vi "SQLite Editing Tests.vi"(8 "Error In (no error)":errorcluster) -> (0 "Error Out":errorcluster)   [LabVIEW 2023]
uses:
  SQLite DB Operator/SQLite DB Operator.lvclass
  H:/Desktop/LabVIEW/LabView Repo/Expenses-Tracker-DB-Operator/DB Operator/DB Operator.lvclass
  SQLite DB Operator/SQLite DB Operator.lvclass/SQLite DB Operator.ctl
  <vilib>/drjdpowell/SQLite Library/SQL Connection/Execute SQL (No results).vi
  <vilib>/drjdpowell/SQLite Library/SQL Connection/Connection.lvclass
  <vilib>/drjdpowell/SQLite Library/SQLite.lvlib
  <vilib>/addons/_JKI Toolkits/Caraya/classes/Test/Test.lvclass
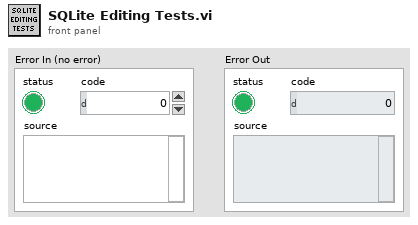
[diagram p1: front panel]
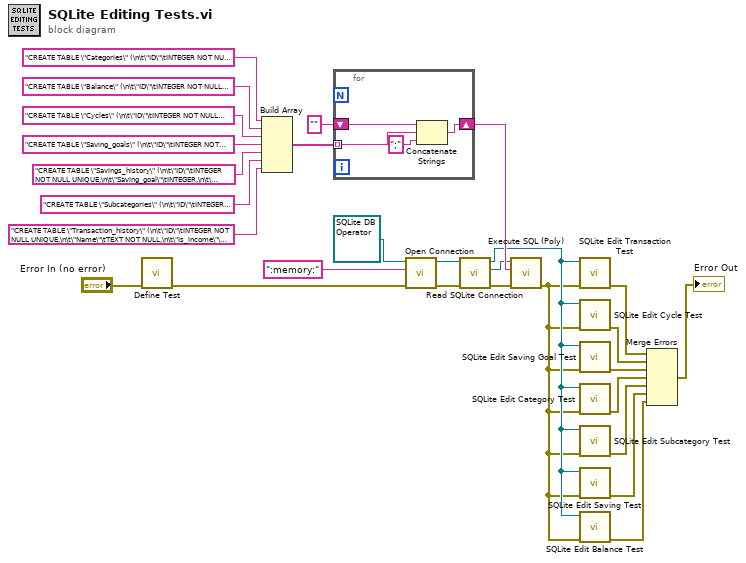
[diagram p0: block diagram]
diagram:
  n1 = call <vilib>:"Define Test.vi"("error in (no error)"="Error In (no error)") -> ("error out"=w11:errorcluster)  [unwired: 9 in, 1 out]
  n2 = Build Array("CREATE TABLE \"Categories\" (\n\t\"ID\"\tINTEGER NOT NULL UNIQUE,\n\t\"Name\"\tTEXT,\n\tPRIMARY KEY(\"ID\" AUTOINCREMENT)\n)", "CREATE TABLE \"Balance\" (\n\t\"ID\"\tINTEGER NOT NULL UNIQUE,\n\t\"Value\"\tREAL NOT NULL,\n\t\"Last_update\"\tINTEGER NOT NULL,\n\tPRIMARY KEY(\"ID\" AUTOINCREMENT)\n)", "CREATE TABLE \"Cycles\" (\n\t\"ID\"\tINTEGER NOT NULL UNIQUE,\n\t\"Name\"\tTEXT,\n\t\"Day_of_occurence\"\tINTEGER,\n\t\"Description\"\tTEXT,\n\tPRIMARY KEY(\"ID\" AUTOINCREMENT)\n)", "CREATE TABLE \"Saving_goals\" (\n\t\"ID\"\tINTEGER NOT NULL UNIQUE,\n\t\"Is_active\"\tINTEGER NOT NULL,\n\t\"Name\"\tTEXT,\n\t\"Current_value\"\tREAL NOT NULL,\n\t\"Target_value\"\tREAL NOT NULL,\n\t\"Date_of_entry\"\tINTEGER NOT NULL,\n\t\"Due_date\"\tINTEGER,\n\t\"Last_update\"\tINTEGER NOT NULL,\n\t\"Description\"\tTEXT,\n\tPRIMARY KEY(\"ID\" AUTOINCREMENT)\n)", "CREATE TABLE \"Savings_history\" (\n\t\"ID\"\tINTEGER NOT NULL UNIQUE,\n\t\"Saving_goal\"\tINTEGER,\n\t\"Value\"\tINTEGER NOT NULL,\n\t\"Date_of_entry\"\tINTEGER NOT NULL,\n\t\"Description\"\tTEXT,\n\tFOREIGN KEY(\"Saving_goal\") REFERENCES \"Saving_goals\"(\"ID\") ON DELETE RESTRICT,\n\tPRIMARY KEY(\"ID\" AUTOINCREMENT)\n)", "CREATE TABLE \"Subcategories\" (\n\t\"ID\"\tINTEGER NOT NULL UNIQUE,\n\t\"Name\"\tTEXT,\n\t\"Category\"\tINTEGER,\n\tFOREIGN KEY(\"Category\") REFERENCES \"Categories\"(\"ID\") ON DELETE SET NULL,\n\tPRIMARY KEY(\"ID\" AUTOINCREMENT)\n)", "CREATE TABLE \"Transaction_history\" (\n\t\"ID\"\tINTEGER NOT NULL UNIQUE,\n\t\"Name\"\tTEXT NOT NULL,\n\t\"Is_income\"\tINTEGER NOT NULL,\n\t\"Value\"\tREAL NOT NULL,\n\t\"Amount\"\tREAL NOT NULL,\n\t\"Total\" REAL GENERATED ALWAYS AS (Amount*Value) STORED,\n\t\"Date_of_entry\"\tINTEGER NOT NULL,\n\t\"Date\"\tINTEGER,\n\t\"Last_update\"\tINTEGER NOT NULL,\n\t\"Category\"\tINTEGER,\n\t\"Subcategory\"\tINTEGER,\n\t\"Cycle\"\tINTEGER,\n\t\"Description\"\tTEXT,\n\tPRIMARY KEY(\"ID\" AUTOINCREMENT),\n\tFOREIGN KEY(\"Cycle\") REFERENCES \"Cycles\"(\"ID\") ON DELETE SET NULL,\n\tFOREIGN KEY(\"Category\") REFERENCES \"Categories\"(\"ID\") ON DELETE SET NULL,\n\tFOREIGN KEY(\"Subcategory\") REFERENCES \"Subcategories\"(\"ID\") ON DELETE SET NULL\n)") -> (w25:string[])
  n3 = for {
    tunnel: w25 -> [w32] mode=indexing
    shift-right: [w30] -> w27
    shift-left: "" -> [w29]
    n4 = Concatenate Strings(w29, w32, ";" ("string")) -> (w30:string)
  }
  n5 = call-dynamic "Open Connection.vi"("Error In (no error)"=w11, "DB Connection String/Path"=":memory:" ("db file"), "SQLite DB Operator In"=refnum<class "SQLite DB Operator.lvclass"> refnum ("SQLite DB Operator.lvclass")) -> ("Error Out"=w15:errorcluster, "SQLite DB Operator Out"=w14:refnum<class "SQLite DB Operator.lvclass">)  [unwired: 7 in]
  n6 = call "Read SQLite Connection.vi"("Error In (no error)"=w15, "SQLite DB Operator In"=w14) -> ("Error Out"=w28:errorcluster, "SQLite.lvlib:Connection"=w16:refnum<class "Connection.lvclass">, "SQLite DB Operator out"=w3:refnum<class "SQLite DB Operator.lvclass">)  [unwired: 7 in]
  n7 = call-poly <vilib>:"Execute SQL (Poly).vi"("error in (no error)"=w28, "SQL"=w27, "SQLite Connection in"=w16) -> ("error out"=w2:errorcluster)  [unwired: 7 in, 1 out]
  n8 = call "SQLite Edit Transaction Test.vi"("Error In (no error)"=w2, "DB Operator In"=w3) -> ("Error Out"=w10:errorcluster)  [unwired: 8 in, 1 out]
  n9 = call "SQLite Edit Cycle Test.vi"("Error In (no error)"=w2, "DB Operator In"=w3) -> ("Error Out"=w9:errorcluster)  [unwired: 8 in, 1 out]
  n10 = call "SQLite Edit Saving Goal Test.vi"("Error In (no error)"=w2, "DB Operator In"=w3) -> ("Error Out"=w8:errorcluster)  [unwired: 8 in, 1 out]
  n11 = call "SQLite Edit Category Test.vi"("Error In (no error)"=w2, "DB Operator In"=w3) -> ("Error Out"=w7:errorcluster)  [unwired: 8 in, 1 out]
  n12 = call "SQLite Edit Subcategory Test.vi"("Error In (no error)"=w2, "DB Operator In"=w3) -> ("Error Out"=w6:errorcluster)  [unwired: 8 in, 1 out]
  n13 = call "SQLite Edit Saving Test.vi"("Error In (no error)"=w2, "DB Operator In"=w3) -> ("Error Out"=w5:errorcluster)  [unwired: 8 in, 1 out]
  n14 = call "SQLite Edit Balance Test.vi"("Error In (no error)"=w2, "DB Operator In"=w3) -> ("Error Out"=w1:errorcluster)  [unwired: 8 in, 1 out]
  n15 = Merge Errors(w10, w9, w8, w7, w6, w5, w1) -> (→"Error Out":errorcluster)
